vi "Modify RT INI.vi"(4 "User defined local path":path, 6 "Keep local copy? (false)":bool, 8 "error in (no error)":errorcluster, 10 "Keys to edit":T1[](array[typedef]), 11 "RT Management in":refnum<class "RT Management.lvclass">) -> (0 "error out":errorcluster, 3 "RT Management out":refnum<class "RT Management.lvclass">)   [LabVIEW 2015, in "RT Management.lvlib" / "RT Management.lvclass"]
doc: "Gets the RT INI file, places it locally, modifies it according to the given \"Keys to edit\", then puts the file back on the RT target. This VI does not restart the target.\n\nThe local file is deleted unless the Keep local copy option is set to true. If so, the user must provide a directory since the default directory is an application specific temporary directory."
uses:
  RT Management.lvclass
  controls/INI key.ctl
  RT Management.lvlib
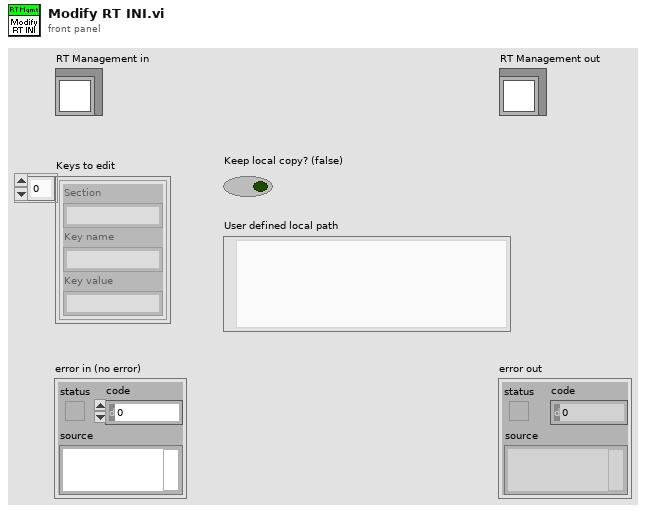
[diagram p1: front panel]
types:
  T1 = typedef "RT Management.lvlib/INI key.ctl" = cluster{"Section":string, "Key name":string, "Key value":string}
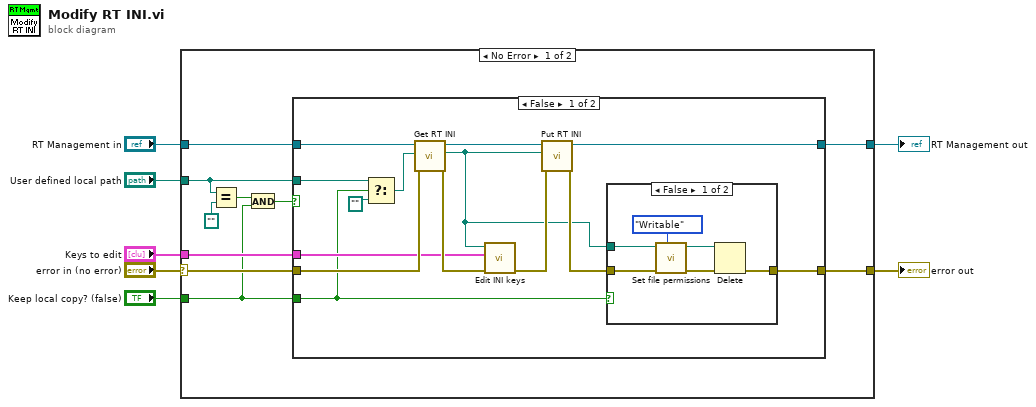
[diagram p0: block diagram]
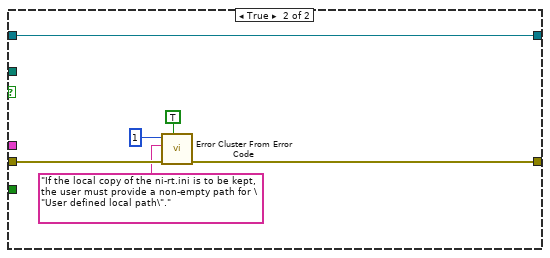
[diagram p3: hidden frame]
diagram:
  n1 = case shown="No Error" "error in (no error)" {
    selector: "error in (no error)" -> [w17 w46]
    tunnel: [w9 w45] -> w5
    tunnel: "RT Management in" -> [w10 w45]
    tunnel: "Keys to edit" -> [w16 _]
    tunnel: [w8 w46] -> w3
    tunnel: "Keep local copy? (false)" -> [w13 _]
    tunnel: "User defined local path" -> [w11 _]
    frame No Error {
      n2 = Equal?(x=w11, y=path "") -> (x = y?=w14:bool)
      n3 = And(x=w14, y=w13) -> (x .and. y?=w12:bool)
      n4 = case shown="False" w12 {
        tunnel: w10 -> [w31 w44]
        tunnel: w17 -> [w30 w42]
        tunnel: w16 -> [w27 _]
        tunnel: [w25 w43] -> w8
        tunnel: [w23 w44] -> w9
        tunnel: w13 -> [w21 _]
        tunnel: w11 -> [w20 _]
        frame False {
          n5 = Select(t=w20, s=w21, f=path "") -> (s? t:f=w18:path)
          n6 = call "Get RT INI.vi"("error in (no error)"=w30, "Non-default local path"=w18, "RT Management in"=w31) -> ("error out"=w28:errorcluster, "Local RT INI path"=w22:path, "RT Management out"=w29:refnum<class "RT Management.lvclass">)  [unwired: 6 in]
          n7 = call "Edit INI keys.vi"("error in (no error)"=w28, "Keys to edit"=w27, "INI file path"=w22) -> ("error out"=w26:errorcluster)  [unwired: 7 in, 1 out]
          n8 = call "Put RT INI.vi"("error in (no error)"=w26, "Local RT INI path"=w22, "RT Management in"=w29) -> ("error out"=w24:errorcluster, "RT Management out"=w23:refnum<class "RT Management.lvclass">)  [unwired: 7 in]
          n9 = case shown="False" w21 {
            tunnel: [w37 w38] -> w25
            tunnel: w24 -> [w33 w38]
            tunnel: w22 -> [w32 _]
            frame False {
              n10 = call "Set file permissions.vi"("Permissions (Writable)"=enum16{"Writable", "Read Only"}."Writable", "error in"=w33, "Path"=w32) -> ("error out"=w36:errorcluster, "Path Out"=w35:path)  [unwired: 7 in]
              n11 = Delete(path (use dialog)=w35, error in=w36) -> (error out=w37:errorcluster)  [unwired: 3 in, 2 out]
            }
            frame True {
            }
          }
        }
        frame True {
          n12 = call <vilib>:"Error Cluster From Error Code.vi"("show call chain? (False)"=TRUE, "error in (no error)"=w42, "error message (\"\")"="If the local copy of the ni-rt.ini is to be kept, the user must provide a non-empty path for \"User defined local path\"." ("error message (\"\")"), "error code (0)"=1) -> ("error out"=w43:errorcluster)  [unwired: 5 in]
        }
      }
    }
    frame Error {
    }
  }
  "error out" <- w3
  "RT Management out" <- w5
